vi "LibXML_EditXML.vi"(6 "mode":T3(ring), 8 "error in":errorcluster, 9 "XML-tree":T1[](array[typedef]), 10 "node":u32, 11 "doc":u32) -> (0 "error out":errorcluster, 1 "first written node":u32, 2 "node copy out":u32, 3 "doc copy out":u32)   [LabVIEW 2019, in "Tools.lvlib" / "LibXML.lvlib"]
doc: "There are 4 edit-modes:\n1. Remove the node from the document\n2. Insert the XML-tree into the document as a child of the selected node\n3. Insert the XML-tree into the document as a sybling of the selected node\n4. Replace the selected node by the XML-tree in the document."
uses:
  LibXML.lvlib
  LibXML_Element.ctl
  LibXML_Attribute.ctl
  LibXML_NavigateDirection.ctl
panel:
  # "This software is FREE licensed under the GNU Lesser General Public License (see license.txt)."
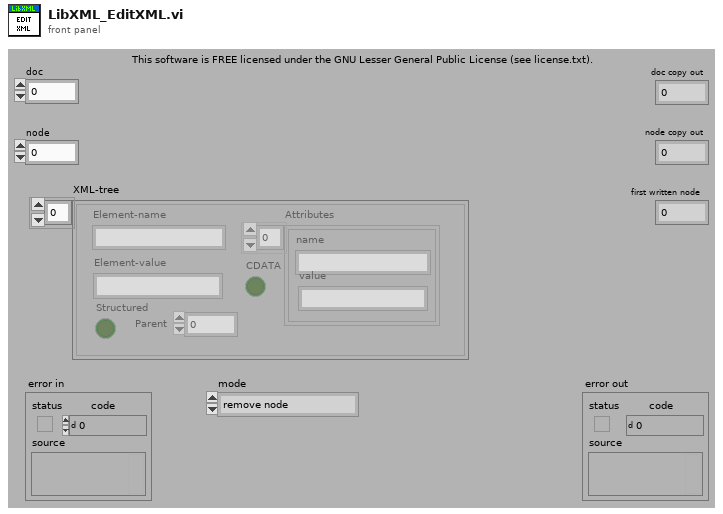
[diagram p1: front panel]
types:
  T1 = typedef "Tools.lvlib/LibXML.lvlib/LibXML_Element.ctl" = cluster{"Element-name":string, "Attributes":T2[], "Element-value":string, "CDATA":bool, "Parent":i32, "Structured":bool}
  T2 = typedef "Tools.lvlib/LibXML.lvlib/LibXML_Attribute.ctl" = cluster{"name":string, "value":string}
  T3 = enum16{"remove node", "replace node", "insert node after", "add new childnode"}
  T4 = typedef "Tools.lvlib/LibXML.lvlib/LibXML_NavigateDirection.ctl" = enum16{"NOP", "first child", "last child", "parent", "next", "prev"}
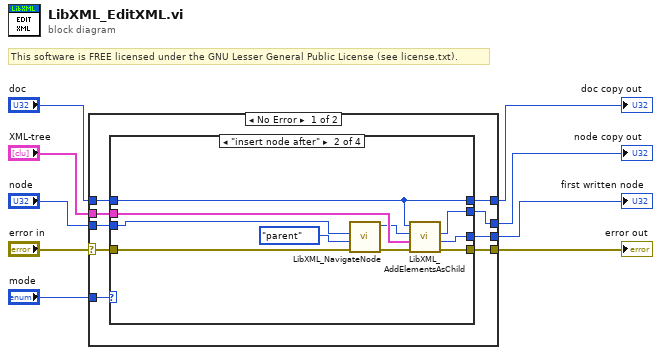
[diagram p0: block diagram]
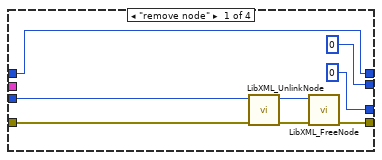
[diagram p2: hidden frame]
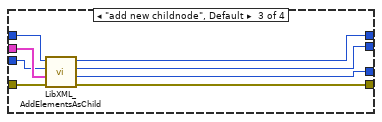
[diagram p3: hidden frame]
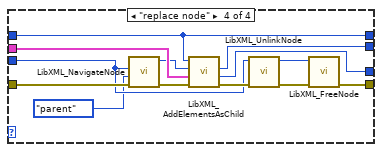
[diagram p4: hidden frame]
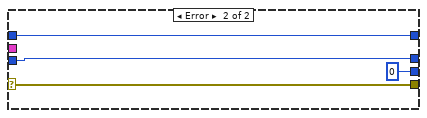
[diagram p5: hidden frame]
diagram:
  # "This software is FREE licensed under the GNU Lesser General Public License (see license.txt)."
  n1 = case shown="No Error" "error in" {
    selector: "error in" -> [w18 w61]
    tunnel: [w16 w61] -> w9
    tunnel: "doc" -> [w17 w60]
    tunnel: "node" -> [w15 w59]
    tunnel: [w14 w60] -> w5
    tunnel: [w13 w59] -> w4
    tunnel: [w12 u32 0 ("first written node")] -> w3
    tunnel: "XML-tree" -> [w11 _]
    tunnel: "mode" -> [w10 _]
    frame No Error {
      n2 = case shown="\"insert node after\"" w10 {
        tunnel: w18 -> [w22 w33 w44 w49]
        tunnel: [w23 w36 w43 w55] -> w16
        tunnel: w11 -> [_ w34 w42 w57]
        tunnel: w17 -> [w26 w35 w41 w56]
        tunnel: w15 -> [w21 w31 w40 w48]
        tunnel: [w26 w35 w39 w56] -> w14
        tunnel: [u32 0 ("parent copy out") w30 w38 w51] -> w13
        tunnel: [u32 0 ("parent copy out") w27 w37 w46] -> w12
        frame "remove node" {
          n3 = call "LibXML_UnlinkNode.vi"("error in"=w22, "node"=w21) -> ("error out"=w25:errorcluster, "node copy out"=w24:u32)  [unwired: 8 in]
          n4 = call "LibXML_FreeNode.vi"("error in"=w25, "node"=w24) -> ("error out"=w23:errorcluster)  [unwired: 9 in]
        }
        frame "insert node after" {
          n5 = call "LibXML_NavigateNode.vi"("error in (no error)"=w33, "direction"=LibXML_NavigateDirection."parent", "node in"=w31) -> ("error out"=w32:errorcluster, "node out"=w29:u32)  [unwired: 2 in, 1 out]
          n6 = call "LibXML_AddElementsAsChild.vi"("error in"=w32, "XML-tree"=w34, "parent"=w29, "doc"=w35) -> ("error out"=w36:errorcluster, "first written node"=w27:u32, "parent copy out"=w30:u32)  [unwired: 4 in, 1 out]
        }
        frame "add new childnode", Default {
          n7 = call "LibXML_AddElementsAsChild.vi"("error in"=w44, "XML-tree"=w42, "parent"=w40, "doc"=w41) -> ("error out"=w43:errorcluster, "first written node"=w37:u32, "parent copy out"=w38:u32, "doc copy out"=w39:u32)  [unwired: 4 in]
        }
        frame "replace node" {
          n8 = call "LibXML_NavigateNode.vi"("error in (no error)"=w49, "direction"=LibXML_NavigateDirection."parent", "node in"=w48) -> ("error out"=w50:errorcluster, "node out"=w45:u32)  [unwired: 2 in, 1 out]
          n9 = call "LibXML_AddElementsAsChild.vi"("error in"=w50, "XML-tree"=w57, "parent"=w45, "doc"=w56) -> ("error out"=w54:errorcluster, "first written node"=w46:u32, "parent copy out"=w51:u32)  [unwired: 4 in, 1 out]
          n10 = call "LibXML_UnlinkNode.vi"("error in"=w54, "node"=w48) -> ("error out"=w53:errorcluster, "node copy out"=w52:u32)  [unwired: 8 in]
          n11 = call "LibXML_FreeNode.vi"("error in"=w53, "node"=w52) -> ("error out"=w55:errorcluster)  [unwired: 9 in]
        }
      }
    }
    frame Error {
    }
  }
  "error out" <- w9
  "doc copy out" <- w5
  "node copy out" <- w4
  "first written node" <- w3
